vi "MasterStateController.vi"(1 "Master State In":T1(ring)) -> (0 "Master State Out":T1(ring))   [LabVIEW 2020]
doc: "This is the master robot state controller. The master robot state can affect any of the subsystem state controllers. Inter-system operations such as end-game sequencers should go here."
uses:
  dsdata.vi
  outputs.vi
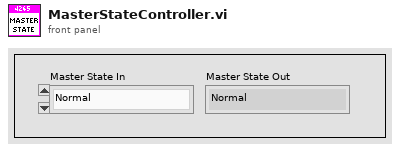
[diagram p1: front panel]
types:
  T1 = enum16{"Normal", "Control Rotation", "Control Position", "Climb"}
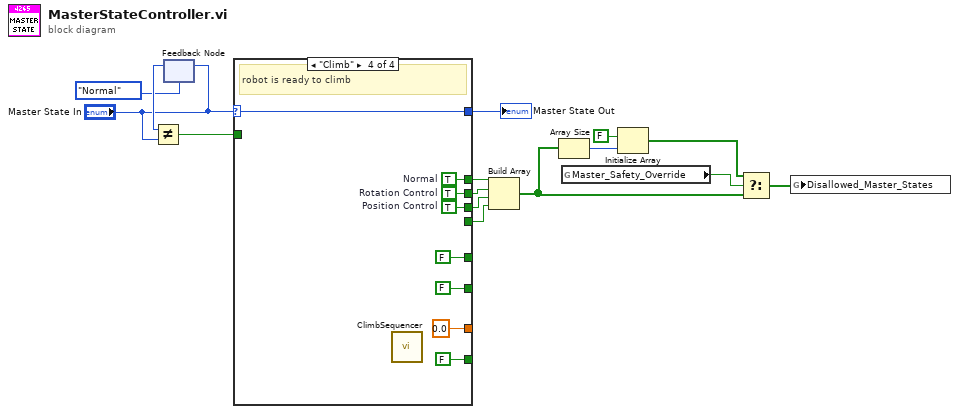
[diagram p0: block diagram]
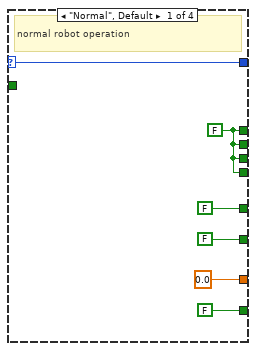
[diagram p2: hidden frame]
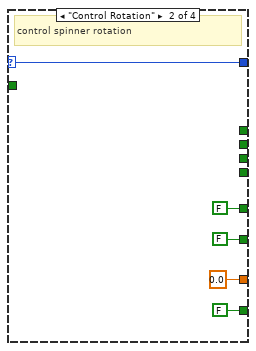
[diagram p3: hidden frame]
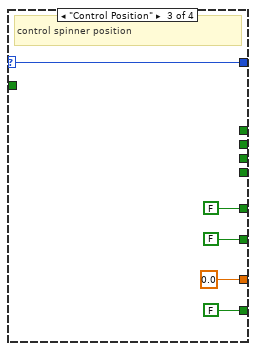
[diagram p4: hidden frame]
diagram:
  n1 = feedback-in #1("Master State In") -> ()
  n2 = feedback #1(T1."Normal" ("Master State In")) -> (w14:T1)
  n3 = Not Equal?(x=w14, y="Master State In") -> (x != y?=w13:bool)
  n4 = case shown="\"Climb\"" "Master State In" {
    selector: "Master State In" -> [w21 w26 w31 w39]
    tunnel: [w21 w26 w31 w39] -> w10
    tunnel: w13 -> [_ _ _ _]
    tunnel: [FALSE ("PTO") FALSE ("PTO") FALSE ("PTO") FALSE ("PTO")] -> _
    tunnel: [FALSE ("Climber Pin") FALSE ("Climber Pin") FALSE ("Climber Pin") FALSE ("Climber Pin")] -> _
    tunnel: [0.0 ("Climber Power") 0.0 ("Climber Power") 0.0 ("Climber Power") 0.0 ("Climber Power")] -> _
    tunnel: [FALSE ("Climber Climbing") FALSE ("Climber Climbing") FALSE ("Climber Climbing") FALSE ("Climber Climbing")] -> _
    tunnel: [w16 _ _ w38] -> w5
    tunnel: [w16 _ _ w37] -> w4
    tunnel: [w16 _ _ w36] -> w3
    tunnel: [w16 _ _ _] -> w2
    frame "Normal", Default {
      w16 = FALSE ("Normal")
      # "normal robot operation"
    }
    frame "Control Rotation" {
      # "control spinner rotation"
    }
    frame "Control Position" {
      # "control spinner position"
    }
    frame "Climb" {
      w37 = TRUE  # Rotation Control
      w36 = TRUE  # Position Control
      w38 = TRUE  # Normal
      # "robot is ready to climb"
      n5 = call "ClimbSequencer.vi"() -> ()  [unwired: 12 in]
    }
  }
  "Master State Out" <- w10
  n6 = Build Array(w5, w4, w3, w2) -> (w6:bool[])
  n7 = Array Size(array=w6) -> (size(s)=w9:i32)
  n8 = global read "dsdata.vi" "Master_Safety_Override"() -> (w15:bool)
  n9 = Initialize Array(FALSE ("element"), w9) -> (w7:bool[])
  n10 = Select(t=w7, s=w15, f=w6) -> (s? t:f=w12:bool[])
  n11 = global write "outputs.vi" "Disallowed_Master_States"(w12) -> ()
